vi "Extract set of 2-port s-parameters from snp-file.vi"() -> ()   [LabVIEW 2020]
uses:
  <vilib>/addons/HF Network Analysis/Support VIs/Read SnP File (SnP).vi
  <vilib>/addons/HF Network Analysis/NI_HFNetworkAnalysis.lvlib
panel:
  in  "Tab Control":enum32{"SP4T", "HFSS"}(tab)
  in  "Test-side row#":i32=16
  in  "Device name offset":i32=27
  in  "\"Device:\" -index":i32=12
  in  "Swap s2p ports":bool=TRUE
  out "New s-parameters":cdb[][](array[numeric])
  out "Comment lines":string[](array[string])
  out "size(s)":i32[](array[numeric])
  out "Original S-parameters":cdb[][](array[numeric]) format="%#.6g"
  in  "Error In":errorcluster
  in  "Swap Ports (False)":bool
  in  "SnP File Path":path
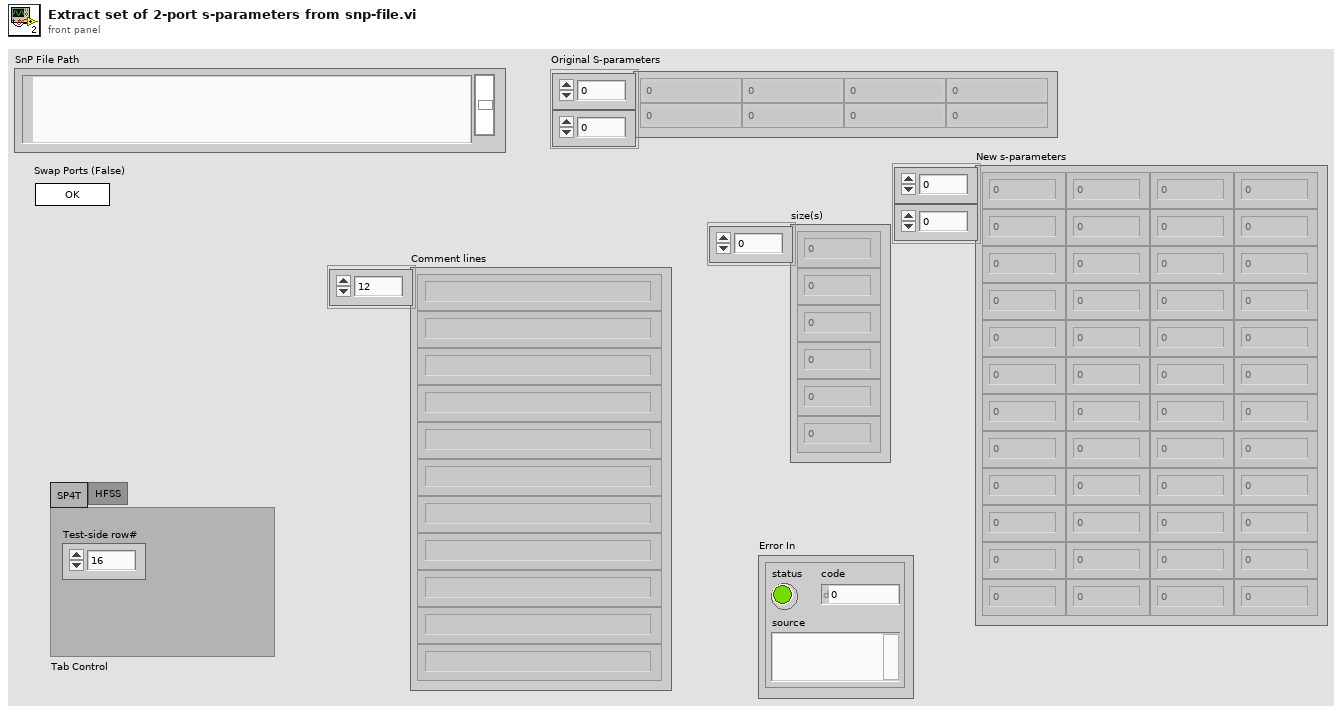
[diagram p1: front panel]
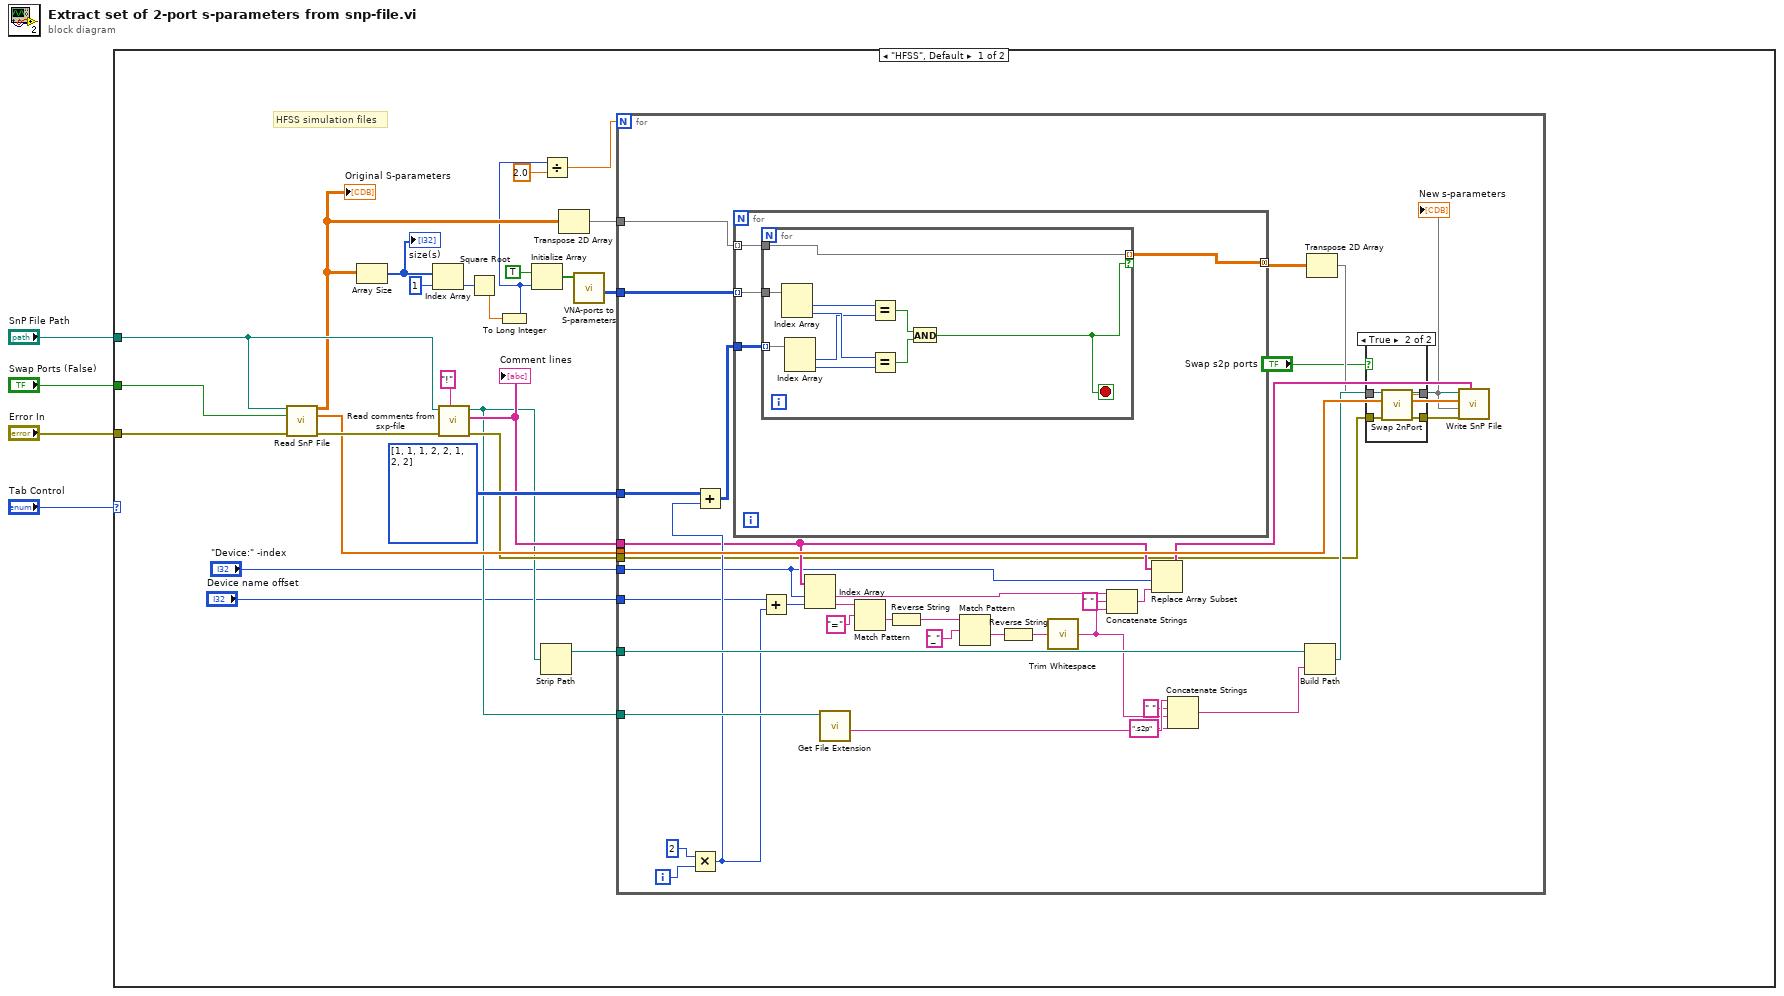
[diagram p0: block diagram]
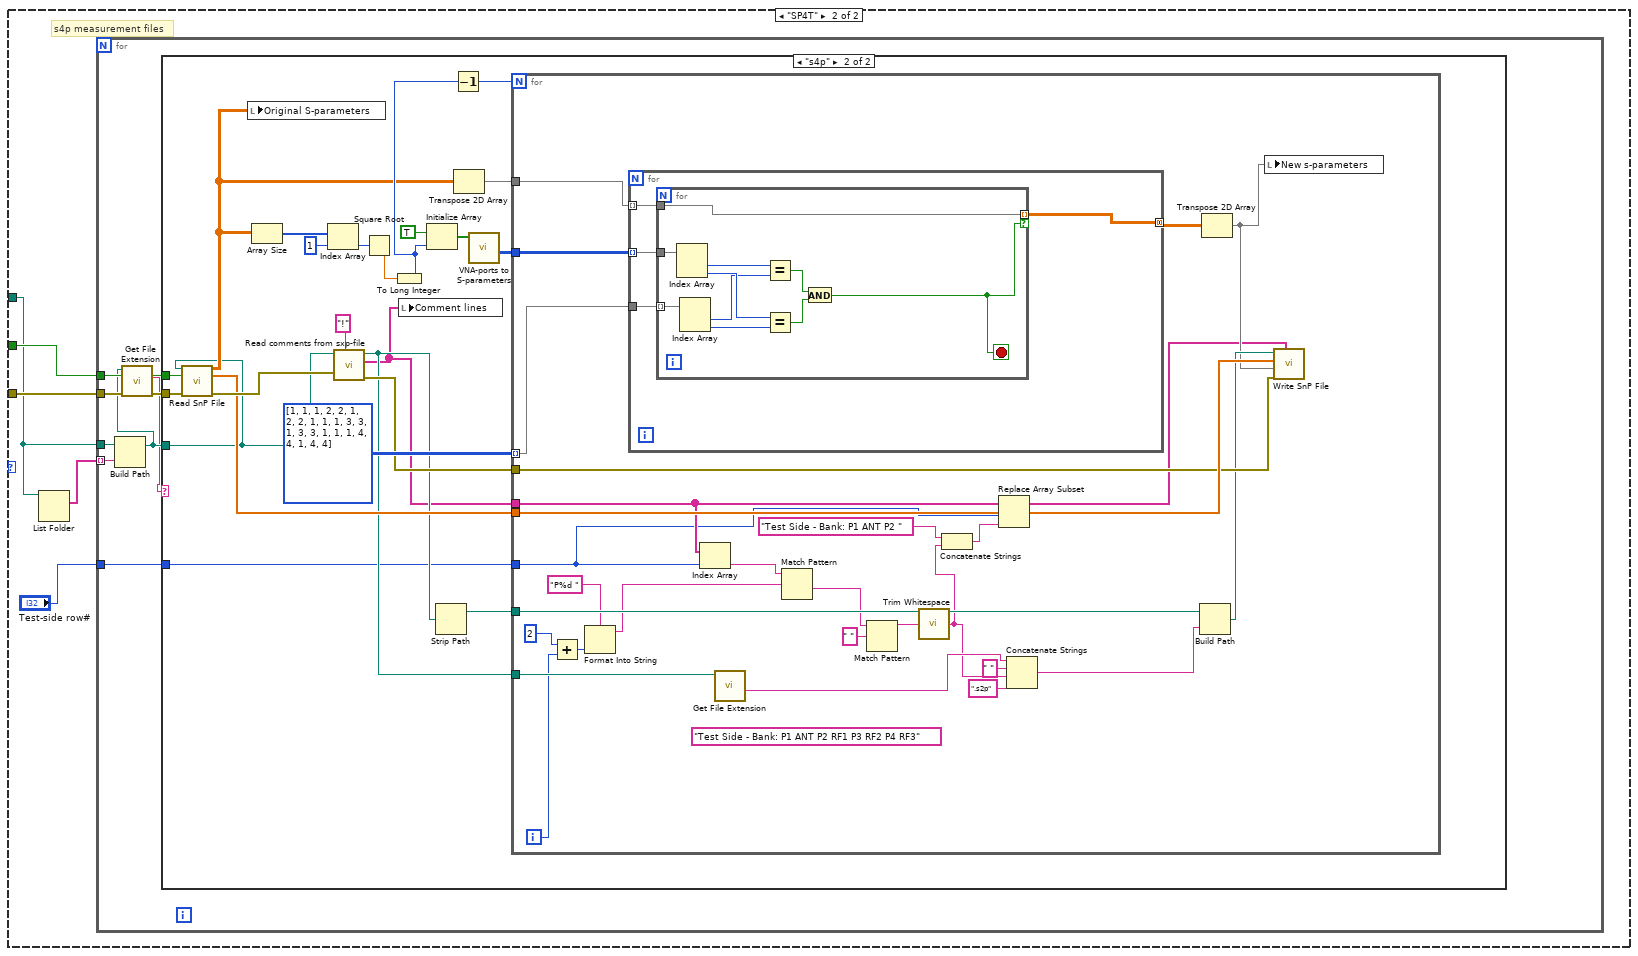
[diagram p3: hidden frame]
diagram:
  n1 = case shown="\"HFSS\", Default" "Tab Control" {
    tunnel: "Swap Ports (False)" -> [w29 w91]
    tunnel: "Error In" -> [w28 w90]
    tunnel: "SnP File Path" -> [w22 w89]
    frame "HFSS", Default {
      # "HFSS simulation files"
      n2 = call-poly <vilib>:"Read SnP File.vi"("SnP File Path"=w22, "Swap Ports (False)"=w29, "Error In"=w28) -> ("S-parameters"=w17:cdb[][], "Frequencies (Hz)"=w15:dbl[], "Error Out"=w20:errorcluster)  [unwired: 9 in, 1 out]
      "Original S-parameters" <- w17
      n3 = Array Size(array=w17) -> (size(s)=w25:i32[])
      "size(s)" <- w25
      n4 = Index Array(array=w25, index=1) -> (element=w24:i32)
      n5 = call "Read comments from sxp-file.vi"("Comment character"="!", "error in (no error)"=w20, "file path"=w22) -> ("error out"=w13:errorcluster, "Comment lines"=w14:string[], "file path out"=w12:path)  [unwired: 6 in]
      "Comment lines" <- w14
      n6 = Square Root(x=w24) -> (sqrt(x)=w8:dbl)
      n7 = To Long Integer(number=w8) -> (32bit integer=w7:i32)
      n8 = Initialize Array(TRUE, w7) -> (w26:bool[])
      n9 = Strip Path(path=w12) -> (stripped path=w11:path)  [unwired: 1 out]
      n10 = Divide(x=w7, y=2.0) -> (x/y=w9:dbl)
      n11 = Transpose 2D Array(2D array=w17) -> (transposed array=w16:cdb[][])
      n12 = call "VNA-ports to S-parameters.vi"("VNA ports"=w26) -> ("Sparameters (ports)"=w19:i32[][])  [unwired: 6 in, 4 out]
      n13 = for {
        N: w9 -> [_]
        tunnel: w19 -> [w66]
        tunnel: i32[][] [[1, 1], [1, 2], [2, 1], [2, 2]] -> [w49]
        tunnel: w16 -> [w65]
        tunnel: w15 -> [w63]
        tunnel: w14 -> [w47]
        tunnel: w13 -> [w34]
        tunnel: w12 -> [w59]
        tunnel: w11 -> [w58]
        tunnel: "\"Device:\" -index" -> [w36]
        tunnel: "Device name offset" -> [w35]
        i -> [w52]
        n14 = Multiply(x=2, y=w52) -> (x*y=w50:i32)
        n15 = Add(x=w49, y=w50) -> (x+y=w48:i32[][])
        n16 = for {
          tunnel: w66 -> [w76] mode=indexing
          tunnel: w65 -> [w75] mode=indexing
          tunnel: w48 -> [w74]
          tunnel: [w73] -> w64 mode=concatenating
          n17 = for {
            tunnel: w76 -> [w86]
            tunnel: w75 -> [w78]
            tunnel: w74 -> [w83] mode=indexing
            tunnel: [w78] -> w73 mode=indexing if=w77
            stop <- w77 stop-if-true
            n18 = Index Array(array=w86) -> (element #1=w85:i32, element #2=w84:i32)  [unwired: 2 in]
            n19 = Index Array(array=w83) -> (element #1=w82:i32, element #2=w81:i32)  [unwired: 2 in]
            n20 = Equal?(x=w85, y=w82) -> (x = y?=w80:bool)
            n21 = Equal?(x=w84, y=w81) -> (x = y?=w79:bool)
            n22 = And(x=w80, y=w79) -> (x .and. y?=w77:bool)
          }
        }
        n23 = Add(x=w35, y=w50) -> (x+y=w53:i32)
        n24 = Index Array(array=w47, index #1=w36, index #2=w53) -> (element #1=w45:string, element #2=w62:string)
        n25 = call <vilib>:"Get File Extension.vi"("file"=w59) -> ("filename without extension"=w57:string)  [unwired: 6 in, 4 out]
        n26 = Match Pattern(string=w62, regular expression="=") -> (after substring=w40:string)  [unwired: 1 in, 3 out]
        n27 = Reverse String(1:w40) -> (0:w39:string)
        n28 = Match Pattern(string=w39, regular expression="_") -> (after substring=w37:string)  [unwired: 1 in, 3 out]
        n29 = Reverse String(1:w37) -> (0:w38:string)
        n30 = call <vilib>:"Trim Whitespace.vi"("string"=w38) -> ("trimmed string"=w43:string)  [unwired: 1 in]
        n31 = Concatenate Strings(w45, " " ("string"), w43) -> (w44:string)
        n32 = Replace Array Subset(array=w47, new element=w44, index=w36) -> (w46:string[])
        n33 = Concatenate Strings(w57, " " ("string"), w43, ".s2p" ("string")) -> (w54:string)
        n34 = Build Path(base path=w58, name or relative path=w54) -> (appended path=w60:path)
        n35 = Transpose 2D Array(2D array=w64) -> (transposed array=w33:cdb[][])
        n36 = case shown="True" "Swap s2p ports" {
          tunnel: w34 -> [w67 w72]
          tunnel: w33 -> [w68 w71]
          tunnel: [w68 w70] -> w32
          tunnel: [w67 w69] -> w30
          frame False {
          }
          frame True {
            n37 = call <vilib>:"Swap 2nPort.vi"("error in (no error)"=w72, "Parameters In (2D)"=w71) -> ("error out"=w69:errorcluster, "Parameters Out (2D)"=w70:cdb[][])  [unwired: 8 in]
          }
        }
        "New s-parameters" <- w32
        n38 = call <vilib>:"Write SnP File.vi"("Comments"=w46, "error in (no error)"=w30, "S-parameters"=w32, "Frequencies (Hz)"=w63, "SnP File Path"=w60) -> ()  [unwired: 6 in, 1 out]
      }
    }
    frame "SP4T" {
      # "s4p measurement files"
      n39 = List Folder(path=w89) -> (filenames=w88:string[])  [unwired: 3 in, 3 out]
      n40 = for {
        tunnel: w91 -> [w99]
        tunnel: w90 -> [w96]
        tunnel: w89 -> [w98]
        tunnel: w88 -> [w97] mode=indexing
        tunnel: "Test-side row#" -> [w92]
        n41 = Build Path(base path=w98, name or relative path=w97) -> (appended path=w94:path)
        n42 = call <vilib>:"Get File Extension.vi"("error in (no error)"=w96, "file"=w94) -> ("error out"=w95:errorcluster, "lowercase file extension"=w93:string)  [unwired: 5 in, 3 out]
        n43 = case shown="\"s4p\"" w93 {
          tunnel: w99 -> [_ w122]
          tunnel: w95 -> [_ w121]
          tunnel: w94 -> [_ w101]
          tunnel: w92 -> [_ w100]
          frame Default {
          }
          frame "s4p" {
            n44 = call-poly <vilib>:"Read SnP File.vi"("SnP File Path"=w101, "Swap Ports (False)"=w122, "Error In"=w121) -> ("S-parameters"=w103:cdb[][], "Frequencies (Hz)"=w110:dbl[], "Error Out"=w114:errorcluster)  [unwired: 9 in, 1 out]
            n45 = local write "Original S-parameters"(w103) -> ()
            n46 = Array Size(array=w103) -> (size(s)=w118:i32[])
            n47 = Index Array(array=w118, index=1) -> (element=w117:i32)
            n48 = call "Read comments from sxp-file.vi"("Comment character"="!", "error in (no error)"=w114, "file path"=w101) -> ("error out"=w109:errorcluster, "Comment lines"=w102:string[], "file path out"=w108:path)  [unwired: 6 in]
            n49 = Square Root(x=w117) -> (sqrt(x)=w105:dbl)
            n50 = To Long Integer(number=w105) -> (32bit integer=w104:i32)
            n51 = local write "Comment lines"(w102) -> ()
            n52 = Initialize Array(TRUE, w104) -> (w119:bool[])
            n53 = Strip Path(path=w108) -> (stripped path=w107:path)  [unwired: 1 out]
            n54 = Decrement(x=w104) -> (x-1=w106:i32)
            n55 = Transpose 2D Array(2D array=w103) -> (transposed array=w111:cdb[][])
            n56 = call "VNA-ports to S-parameters.vi"("VNA ports"=w119) -> ("Sparameters (ports)"=w113:i32[][])  [unwired: 6 in, 4 out]
            n57 = for {
              N: w106 -> [_]
              tunnel: w113 -> [w151]
              tunnel: i32[][][] [[[1, 1], [1, 2], [2, 1], [2, 2]], [[1, 1], [1, 3], [3, 1], [3, 3]], [[1, 1], [1, 4], [4, 1], [4, 4]]] -> [w136] mode=indexing
              tunnel: w111 -> [w150]
              tunnel: w110 -> [w148]
              tunnel: w102 -> [w134]
              tunnel: w109 -> [w146]
              tunnel: w108 -> [w144]
              tunnel: w107 -> [w143]
              tunnel: w100 -> [w123]
              i -> [w137]
              (unwired) "Test Side - Bank: P1 ANT P2 RF1 P3 RF2 P4 RF3" ("regular expression")
              n58 = Add(x=2 ("index"), y=w137) -> (x+y=w131:i32)
              n59 = Format Into String(format string="P%d " ("regular expression"), w131) -> (resulting string=w130:string)  [unwired: 2 in, 1 out]
              n60 = for {
                tunnel: w151 -> [w155] mode=indexing
                tunnel: w150 -> [w154] mode=indexing
                tunnel: w136 -> [w153]
                tunnel: [w152] -> w149 mode=concatenating
                n61 = for {
                  tunnel: w155 -> [w165]
                  tunnel: w154 -> [w157]
                  tunnel: w153 -> [w162] mode=indexing
                  tunnel: [w157] -> w152 mode=indexing if=w156
                  stop <- w156 stop-if-true
                  n62 = Index Array(array=w165) -> (element #1=w164:i32, element #2=w163:i32)  [unwired: 2 in]
                  n63 = Index Array(array=w162) -> (element #1=w161:i32, element #2=w160:i32)  [unwired: 2 in]
                  n64 = Equal?(x=w164, y=w161) -> (x = y?=w159:bool)
                  n65 = Equal?(x=w163, y=w160) -> (x = y?=w158:bool)
                  n66 = And(x=w159, y=w158) -> (x .and. y?=w156:bool)
                }
              }
              n67 = Index Array(array=w134, index=w123) -> (element=w147:string)
              n68 = call <vilib>:"Get File Extension.vi"("file"=w144) -> ("filename without extension"=w142:string)  [unwired: 6 in, 4 out]
              n69 = Match Pattern(string=w147, regular expression=w130) -> (after substring=w128:string)  [unwired: 1 in, 3 out]
              n70 = Match Pattern(string=w128, regular expression=" ") -> (before substring=w127:string)  [unwired: 1 in, 3 out]
              n71 = call <vilib>:"Trim Whitespace.vi"("string"=w127) -> ("trimmed string"=w125:string)  [unwired: 1 in]
              n72 = Concatenate Strings("Test Side - Bank: P1 ANT P2 " ("regular expression"), w125) -> (w124:string)
              n73 = Replace Array Subset(array=w134, new element=w124, index=w123) -> (w133:string[])
              n74 = Concatenate Strings(w142, " " ("string"), w125, ".s2p" ("string")) -> (w139:string)
              n75 = Build Path(base path=w143, name or relative path=w139) -> (appended path=w145:path)
              n76 = Transpose 2D Array(2D array=w149) -> (transposed array=w135:cdb[][])
              n77 = local write "New s-parameters"(w135) -> ()
              n78 = call <vilib>:"Write SnP File.vi"("Comments"=w133, "error in (no error)"=w146, "S-parameters"=w135, "Frequencies (Hz)"=w148, "SnP File Path"=w145) -> ()  [unwired: 6 in, 1 out]
            }
          }
        }
      }
    }
  }
